vi "主程序.vi"() -> ()   [LabVIEW 2010]
panel:
  out "op":string
  out "ans":dbl
  in  "y":dbl
  in  "x":dbl
  in  "?":i8(slide) scale=0.0..3.0
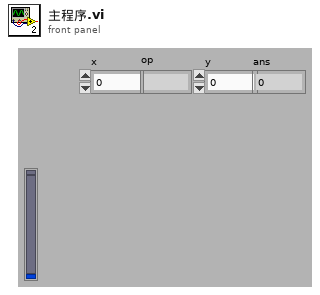
[diagram p1: front panel]
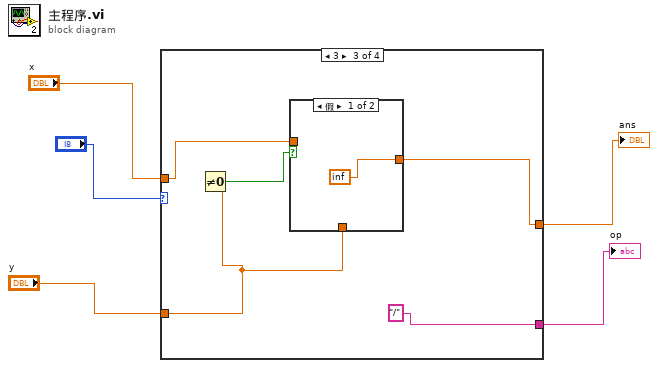
[diagram p0: block diagram]
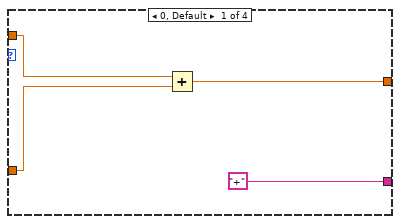
[diagram p2: hidden frame]
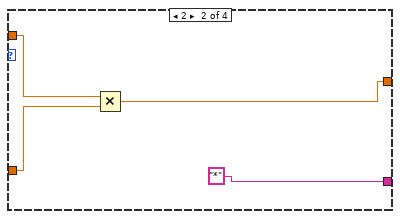
[diagram p3: hidden frame]
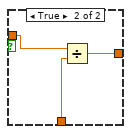
[diagram p4: hidden frame]
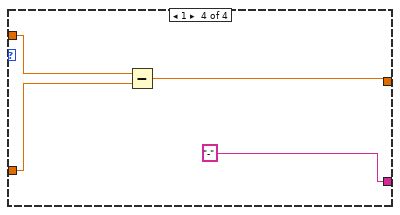
[diagram p5: hidden frame]
diagram:
  n1 = case "条件结构" shown="3" "?" {
    tunnel: "x" -> [w9 w13 w16 w26]
    tunnel: "y" -> [w8 w12 w15 w25]
    tunnel: ["+" "*" "/" "-"] -> w2
    tunnel: [w6 w11 w14 w24] -> w1
    frame 0, Default {
      n2 = Add(x=w9, y=w8) -> (x+y=w6:dbl)
    }
    frame 2 {
      n3 = Multiply(x=w13, y=w12) -> (x*y=w11:dbl)
    }
    frame 3 {
      n4 = Not Equal To 0?(x=w15) -> (x != 0?=w17:bool)
      n5 = case shown="假" w17 {
        tunnel: w16 -> [_ w22]
        tunnel: w15 -> [_ w21]
        tunnel: [inf w20] -> w14
        frame False {
        }
        frame True {
          n6 = Divide(x=w22, y=w21) -> (x/y=w20:dbl)
        }
      }
    }
    frame 1 {
      n7 = Subtract(x=w26, y=w25) -> (x-y=w24:dbl)
    }
  }
  "ans" <- w1
  "op" <- w2
